vi "testOpMux_New.vi"() -> ()   [LabVIEW 2014]
uses:
  Multiplexer_Opmux.lvclass
panel:
  out "Multiplexer_Opmux out":refnum<class "Multiplexer_Opmux.lvclass">
  out "BufferOut":string
  out "DevFound?":bool
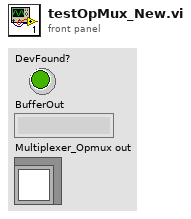
[diagram p1: front panel]
types:
  T1 = enum16{"Version?", "Software Trigger", "Reset", "Radiator Temp?", "In Voltage?"}
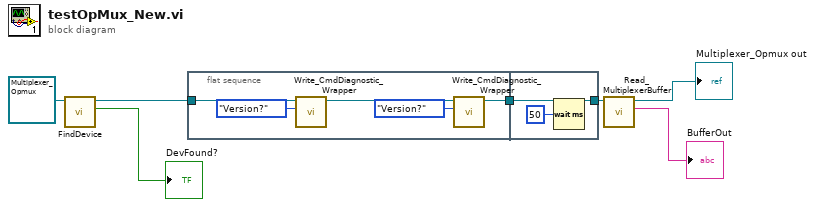
[diagram p0: block diagram]
diagram:
  n1 = call-dynamic "FindDevice.vi"("Multiplexer_Opmux in"=refnum<class "Multiplexer_Opmux.lvclass"> refnum) -> ("DevFound?"=→"DevFound?":bool, "Multiplexer_Opmux out"=w6:refnum<class "Multiplexer_Opmux.lvclass">)  [unwired: 8 in, 1 out]
  n2 = flat-sequence {
    tunnel: w6 -> [w12]
    tunnel: [w8] -> w4
    tunnel: [w14] -> w5
    tunnel: w4 -> [w14]
    frame #0 {
      n3 = call-dynamic "Write_CmdDiagnostic_Wrapper.vi"("Command"=T1."Version?", "Multiplexer_Opmux in"=w12) -> ("Multiplexer_Opmux out"=w10:refnum<class "Multiplexer_Opmux.lvclass">)  [unwired: 8 in, 1 out]
      n4 = call-dynamic "Write_CmdDiagnostic_Wrapper.vi"("Command"=T1."Version?", "Multiplexer_Opmux in"=w10) -> ("Multiplexer_Opmux out"=w8:refnum<class "Multiplexer_Opmux.lvclass">)  [unwired: 8 in, 1 out]
    }
    frame #1 {
      n5 = Wait (ms)(milliseconds to wait=u32 50) -> ()  [unwired: 1 out]
    }
  }
  n6 = call-dynamic "Read_MultiplexerBuffer.vi"("Multiplexer_Opmux in"=w5) -> ("BufferOut"=→"BufferOut":string, "Multiplexer_Opmux out"=→"Multiplexer_Opmux out":refnum<class "Multiplexer_Opmux.lvclass">)  [unwired: 8 in, 1 out]
